vi "Dynamic Channel Global.vi"() -> ()   [LabVIEW 2020]
panel:
  in  "Number of Channels Param Name":string="Number of Channels"
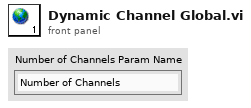
[diagram p1: front panel]
diagram:
